vi "Insert_Fix Node Terminals.vi"(6 "Inserted Node":refnum<vi>, 8 "error in (no error)":errorcluster, 9 "Original Wire":refnum<vi>, 11 "Node Name":string) -> (0 "error out":errorcluster)   [LabVIEW 2017]
doc: "When the LabVIEW Insert algorithm inserts the node in a non-ideal manner on a wire, this VI will fix the wiring in those specific cases."
uses:
  <vilib>/Utility/Data Type/Type Definitions/Data Type.ctl
  <vilib>/Utility/Data Type/NI_Data Type.lvlib
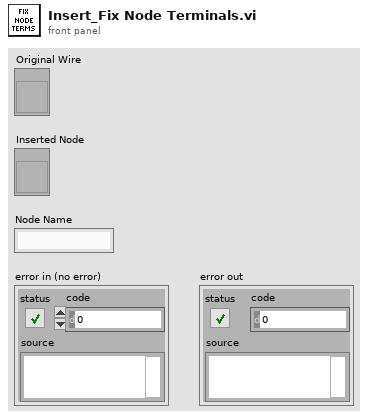
[diagram p1: front panel]
types:
  T1 = typedef "NI_Data Type.lvlib/Data Type.ctl" = enum8{"Invalid Type", "Void", "I8", "I16", "I32", "I64", "U8", "U16", "U32", "U64", "Single Float", "Double Float", "Extended Float", "Single Complex", "Double Complex", "Extended Complex", "Enum U8", "Enum U16", "Enum U32", "Enum U64", "Single Float With Unit", "Double Float With Unit", "Extended Float With Unit", "Single Complex with Unit", "Double Complex with Unit", "Extended Complex with Unit", "Boolean", "String", "Path", "Picture", "Tag", "Array", "Cluster", "Variant", "LV Variant", "Waveform", "Timestamp", "Digital Waveform", "Digital Data", "ExpressData", "Refnum", "External Data", "VI", "Poly VI", "LabVIEW Class Instance", "Fixed Point"}
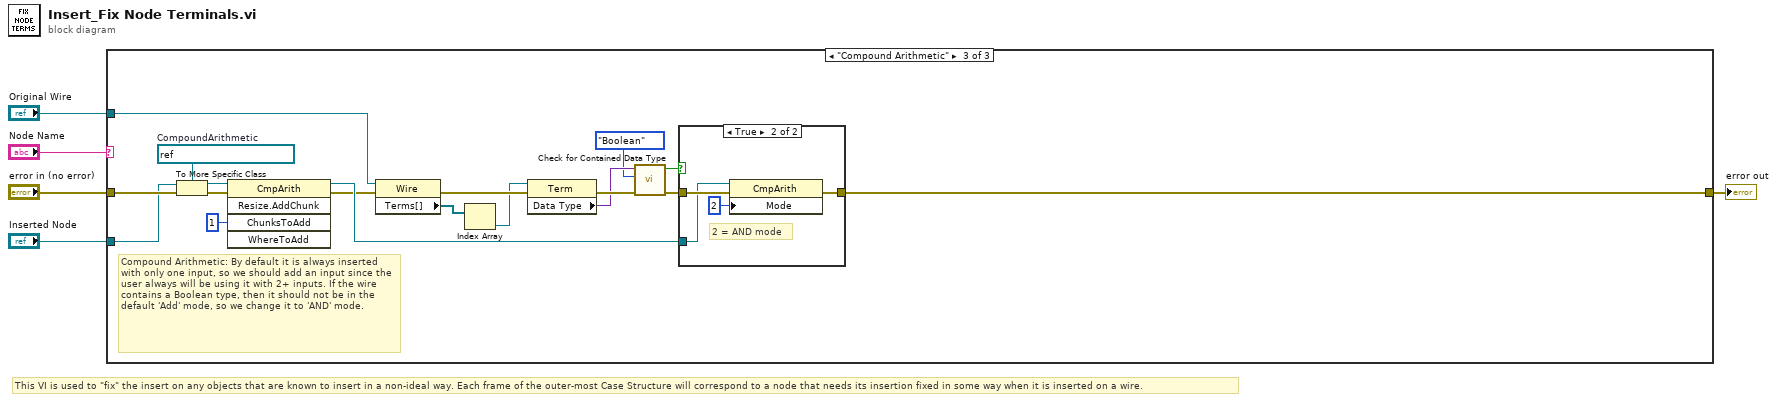
[diagram p0: block diagram]
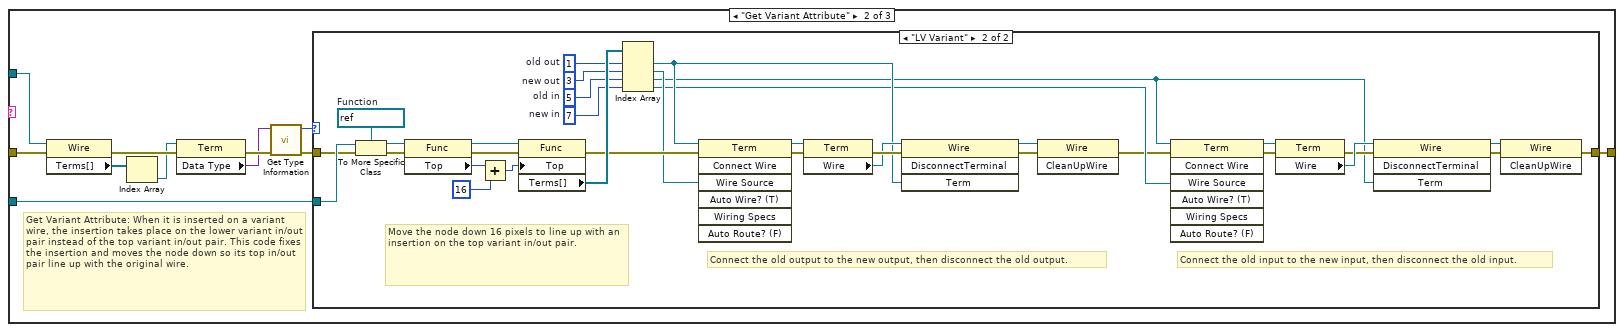
[diagram p3: hidden frame]
diagram:
  # "This VI is used to \"fix\" the insert on any objects that are known to insert in a non-ideal way. Each frame of the outer-most Case Structure will correspond to a node that needs its insertion fixed in some way when it is inserted on a wire."
  n1 = case shown="\"Compound Arithmetic\"" "Node Name" {
    tunnel: "error in (no error)" -> [w6 w17 w58]
    tunnel: [w6 w8 w63] -> w3
    tunnel: "Original Wire" -> [_ w16 w70]
    tunnel: "Inserted Node" -> [_ w7 w57]
    frame Default {
    }
    frame "Get Variant Attribute" {
      # "Get Variant Attribute: When it is inserted on a variant wire, the insertion takes place on the lower variant in/out pair instead of the top variant in/out pair. This code fixes the insertion and moves the node down so its top in/out pair line up with the original wire."
      n2 = property class="Wire"(reference=w16, error in=w17) -> (error out=w14:errorcluster, "Terms[]"=w15:refnum<vi>[])  [unwired: 1 out]
      n3 = Index Array(array=w15) -> (element=w13:refnum<vi>)  [unwired: 1 in]
      n4 = property class="Term"(reference=w13, error in=w14) -> (error out=w12:errorcluster, "Data Type"=w11:variant)  [unwired: 1 out]
      n5 = call <vilib>:"Get Type Information.vi"("error in (no error)"=w12, "Variant"=w11) -> ("error out"=w10:errorcluster, "Type"=w9:T1)  [unwired: 5 in, 3 out]
      n6 = case shown="\"LV Variant\"" w9 {
        tunnel: w10 -> [w18 w50]
        tunnel: [w18 w22] -> w8
        tunnel: w7 -> [_ w52]
        frame Default {
          # "Do nothing if the insert took place on a non-variant wire, like the error cluster."
        }
        frame "LV Variant" {
          w38 = 7  # new in
          w39 = 5  # old in
          w40 = 3  # new out
          w41 = 1  # old out
          w48 = refnum<vi> refnum  # Function
          # "Connect the old input to the new input, then disconnect the old input."
          # "Connect the old output to the new output, then disconnect the old output."
          # "Move the node down 16 pixels to line up with an insertion on the top variant in/out pair."
          n7 = To More Specific Class(target class=w48, reference=w52, error in=w50) -> (specific class reference=w51:refnum<vi>, error out=w49:errorcluster)
          n8 = property class="Func"(reference=w51, error in=w49) -> (reference out=w46:refnum<vi>, error out=w47:errorcluster, "Top"=w45:i32)
          n9 = Add(x=w45, y=16) -> (x+y=w44:i32)
          n10 = property class="Func"(reference=w46, error in=w47, "Top"=w44) -> (error out=w37:errorcluster, "Terms[]"=w42:refnum<vi>[])  [unwired: 1 out]
          n11 = Index Array(array=w42, index #1=w41, index #2=w40, index #3=w39, index #4=w38) -> (element #1=w31:refnum<vi>, element #2=w36:refnum<vi>, element #3=w25:refnum<vi>, element #4=w24:refnum<vi>)
          n12 = invoke class="Term" method="Connect Wire"(reference=w31, error in=w37, "Wire Source"=w36) -> (reference out=w34:refnum<vi>, error out=w35:errorcluster)  [unwired: 4 in, 5 out]
          n13 = property class="Term"(reference=w34, error in=w35) -> (error out=w33:errorcluster, "Wire"=w32:refnum<vi>)  [unwired: 1 out]
          n14 = invoke class="Wire" method="DisconnectTerminal"(reference=w32, error in=w33, "Term"=w31) -> (reference out=w19:refnum<vi>, error out=w26:errorcluster)  [unwired: 1 in, 2 out]
          n15 = invoke class="Wire" method="CleanUpWire"(reference=w19, error in=w26) -> (error out=w20:errorcluster)  [unwired: 1 in, 2 out]
          n16 = invoke class="Term" method="Connect Wire"(reference=w25, error in=w20, "Wire Source"=w24) -> (reference out=w28:refnum<vi>, error out=w27:errorcluster)  [unwired: 4 in, 5 out]
          n17 = property class="Term"(reference=w28, error in=w27) -> (error out=w29:errorcluster, "Wire"=w30:refnum<vi>)  [unwired: 1 out]
          n18 = invoke class="Wire" method="DisconnectTerminal"(reference=w30, error in=w29, "Term"=w25) -> (reference out=w21:refnum<vi>, error out=w23:errorcluster)  [unwired: 1 in, 2 out]
          n19 = invoke class="Wire" method="CleanUpWire"(reference=w21, error in=w23) -> (error out=w22:errorcluster)  [unwired: 1 in, 2 out]
        }
      }
    }
    frame "Compound Arithmetic" {
      w59 = refnum<vi> refnum  # CompoundArithmetic
      # "Compound Arithmetic: By default it is always inserted with only one input, so we should add an input since the user always will be using it with 2+ inputs. If the wire contains a Boolean type, then it should not be in the default 'Add' mode, so we change it to 'AND' mode."
      n20 = To More Specific Class(target class=w59, reference=w57, error in=w58) -> (specific class reference=w61:refnum<vi>, error out=w60:errorcluster)
      n21 = invoke class="CmpArith" method="Resize.AddChunk"(reference=w61, error in=w60, "ChunksToAdd"=u8 1 ("Chunks To Add")) -> (reference out=w56:refnum<vi>, error out=w55:errorcluster)  [unwired: 2 in, 3 out]
      n22 = property class="Wire"(reference=w70, error in=w55) -> (error out=w68:errorcluster, "Terms[]"=w69:refnum<vi>[])  [unwired: 1 out]
      n23 = Index Array(array=w69) -> (element=w67:refnum<vi>)  [unwired: 1 in]
      n24 = property class="Term"(reference=w67, error in=w68) -> (error out=w66:errorcluster, "Data Type"=w65:variant)  [unwired: 1 out]
      n25 = call <vilib>:"Check for Contained Data Type.vi"("error in (no error)"=w66, "Data Type to Find"=Data_Type."Boolean", "Variant"=w65) -> ("error out"=w64:errorcluster, "Contains Data Type to Find?"=w54:bool)  [unwired: 7 in]
      n26 = case shown="True" w54 {
        tunnel: w64 -> [w71 w73]
        tunnel: [w71 w74] -> w63
        tunnel: w56 -> [_ w72]
        frame False {
          # "Wire doesn't contain Boolean, so it's safe to leave CA in 'Add' mode."
        }
        frame True {
          # "2 = AND mode"
          n27 = property class="CmpArith"(reference=w72, error in=w73, "Mode"=u32 2) -> (error out=w74:errorcluster)  [unwired: 1 out]
        }
      }
    }
  }
  "error out" <- w3
